vi "2dlev-mar abx.vi"(0 "X":dbl[](array[numeric]) format="%.2f", 2 "Y":dbl[](array[numeric]) format="%.2f", 3 "Coefficients":dbl[](array[numeric]) format="%.2f", 5 "W":dbl[](array[numeric]) format="%.2f") -> (6 "Alpha":dbl[][](array[numeric]) format="%.2f", 7 "Beta":dbl[](array[numeric]) format="%.2f", 8 "chiSqr":dbl format="%.2f")   [LabVIEW 2009]
panel:
  # "Array Lev-Mar\nabx"
  # "Array modifications by\nChristian Altenbach\ncaltenba@ucla.edu"
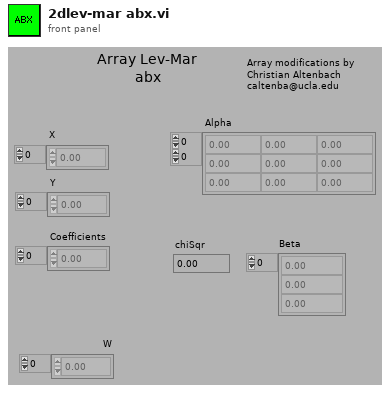
[diagram p1: front panel]
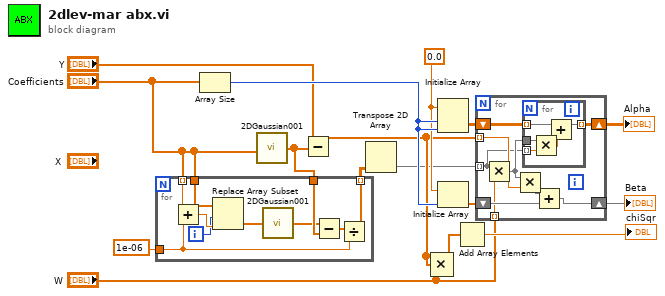
[diagram p0: block diagram]
diagram:
  w13 = 0.0
  n1 = Array Size(array="Coefficients") -> (size(s)=w16:i32)
  n2 = call "2DGaussian001.vi"("Paramters"="Coefficients") -> ("Flattened Image"=w1:dbl[])
  n3 = for {
    tunnel: [w22] -> w3 mode=indexing
    tunnel: "Coefficients" -> [w23] mode=indexing
    tunnel: "Coefficients" -> [w21]
    tunnel: 1e-06 -> [w20]
    tunnel: w1 -> [w19]
    i -> [w24]
    n4 = Add(x=w23, y=w20) -> (x+y=w25:dbl)
    n5 = Replace Array Subset(array=w21, new element=w25, index=w24) -> (w18:dbl[])
    n6 = call "2DGaussian001.vi"("Paramters"=w18) -> ("Flattened Image"=w17:dbl[])
    n7 = Subtract(x=w17, y=w19) -> (x-y=w26:dbl[])
    n8 = Divide(x=w26, y=w20) -> (x/y=w22:dbl[])
  }
  n9 = Subtract(x="Y", y=w1) -> (x-y=w9:dbl[])
  n10 = Transpose 2D Array(2D array=w3) -> (transposed array=w5:dbl[][])
  n11 = Compound Arithmetic op=MULTIPLY(w9, w9, "W") -> (w8:dbl[])
  n12 = Initialize Array(w13, w16, w16) -> (w14:dbl[][])
  n13 = Initialize Array(w13, w16) -> (w15:dbl[])
  n14 = Add Array Elements(numeric array=w8) -> (sum=→"chiSqr":dbl)
  n15 = for {
    shift-right: [w33] -> w12
    shift-left: w15 -> [w35]
    shift-right: [w31] -> w11
    shift-left: w14 -> [w32]
    tunnel: w5 -> [w27] mode=indexing
    tunnel: w9 -> [w30] mode=indexing
    tunnel: "W" -> [w29] mode=indexing
    n16 = Multiply(x=w27, y=w29) -> (x*y=w28:dbl[])
    n17 = Multiply(x=w28, y=w30) -> (x*y=w34:dbl[])
    n18 = for {
      tunnel: w28 -> [w40]
      tunnel: w32 -> [w39] mode=indexing
      tunnel: [w37] -> w31 mode=indexing
      tunnel: w27 -> [w36] mode=indexing
      n19 = Multiply(x=w40, y=w36) -> (x*y=w38:dbl[])
      n20 = Add(x=w39, y=w38) -> (x+y=w37:dbl[])
    }
    n21 = Add(x=w34, y=w35) -> (x+y=w33:dbl[])
  }
  "Alpha" <- w11
  "Beta" <- w12
